vi "WSVCAP SHL Host LL Set Read_Write Parameters.vi"(0 "Transaction":T1, 1 "Wait Ticks":u32, 2 "Slave Address":u8, 5 "Bytes":u8, 7 "Sub Address [U8]":u8=191 format="%.0x", 9 "Socket Mask [U64]":u64=1 format="%016x", 11 "error in (no error)":errorcluster) -> (15 "error out":errorcluster)   [LabVIEW 2012]
uses:
  Type Defs/WSVCAP SHL Transaction Enum.ctl
  Type Defs/WSVCAP SHL Top Level Control Operation Enum.ctl
  Type Defs/WSVCAP SHL State.ctl
  Type Defs/WSVCAP SHL Top Level Control Enum.ctl
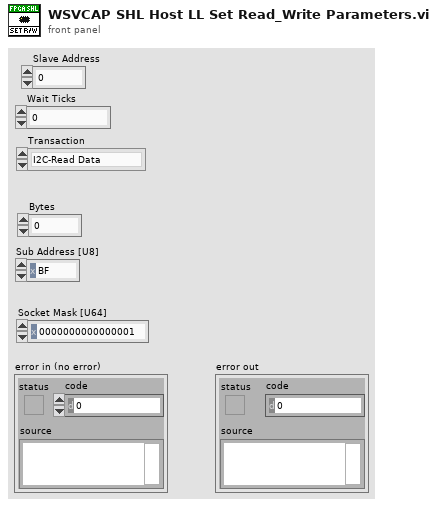
[diagram p1: front panel]
types:
  T1 = typedef "WSVCAP SHL Transaction Enum.ctl" = enum16{"I2C-Read Data", "I2C-Write Data", "SPI-Write/Read Data", "RFFE-Ext Write", "RFFE-Ext Read"}
  T2 = typedef "WSVCAP SHL Top Level Control Enum.ctl" = enum16{"Start", "Cmd", "Transaction", "Wait Ticks", "Socket Mask", "Slave Address", "Sub Address", "Bytes to Write", "Bytes to Read", "Write Data", "Write Flag", "Read Data", "Read Flag", "Ack Read", "Read Status Flag", "Ack Read Status", "Status", "Cycle Count", "Stop Cycle", "Exit"}
  T3 = typedef "WSVCAP SHL State.ctl" = enum8{"Idle", "Transfer Data"}
  T4 = typedef "WSVCAP SHL Top Level Control Operation Enum.ctl" = enum16{"Initialize", "Set Control", "Read Control", "Close"}
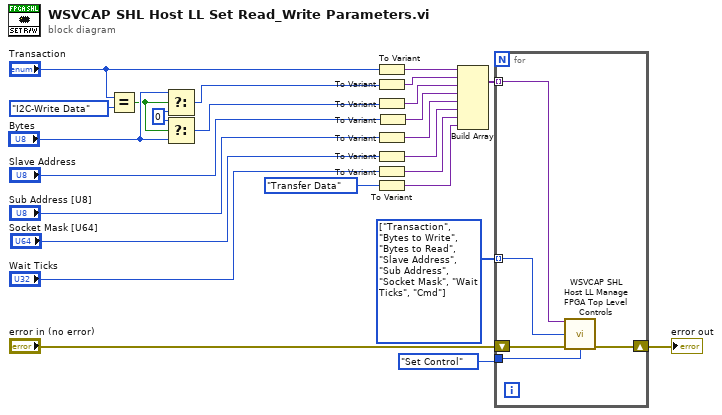
[diagram p0: block diagram]
diagram:
  w16 = u8 0 ("t")
  w18 = T2[] [enum."Transaction", enum."Bytes to Write", enum."Bytes to Read", enum."Slave Address", enum."Sub Address", enum."Socket Mask", enum."Wait Ticks", enum."Cmd"] items=["Start", "Cmd", "Transaction", "Wait Ticks", "Socket Mask", "Slave Address", "Sub Address", "Bytes to Write", "Bytes to Read", "Write Data", "Write Flag", "Read Data", "Read Flag", "Ack Read", "Read Status Flag", "Ack Read Status", "Status", "Cycle Count", "Stop Cycle", "Exit"]
  n1 = Equal?(x="Transaction", y=WSVCAP_SHL_Transaction_Enum."I2C-Write Data" ("Transaction")) -> (x = y?=w10:bool)
  n2 = Select(t="Bytes", s=w10, f=w16) -> (s? t:f=w15:u8)
  n3 = Select(t=w16, s=w10, f="Bytes") -> (s? t:f=w14:u8)
  n4 = To Variant(anything="Transaction") -> (Variant=w24:variant)
  n5 = To Variant(anything=w15) -> (Variant=w23:variant)
  n6 = To Variant(anything=w14) -> (Variant=w13:variant)
  n7 = To Variant(anything="Sub Address [U8]") -> (Variant=w9:variant)
  n8 = To Variant(anything="Socket Mask [U64]") -> (Variant=w8:variant)
  n9 = To Variant(anything="Wait Ticks") -> (Variant=w4:variant)
  n10 = To Variant(anything=WSVCAP_SHL_State."Transfer Data" ("SPI_Cmd")) -> (Variant=w19:variant)
  n11 = To Variant(anything="Slave Address") -> (Variant=w1:variant)
  n12 = Build Array(w24, w23, w13, w1, w9, w8, w4, w19) -> (w22:variant[])
  n13 = for {
    tunnel: WSVCAP_SHL_Top_Level_Control_Operation_Enum."Set Control" ("Operation") -> [w30]
    tunnel: w22 -> [w29] mode=indexing
    tunnel: w18 -> [w28] mode=indexing
    shift-right: [w26] -> w20
    shift-left: "error in (no error)" -> [w27]
    n14 = call "WSVCAP SHL Host LL Manage FPGA Top Level Controls.vi"("Value In"=w29, "FPGA Top Level Control"=w28, "error in (no error)"=w27, "Operation"=w30) -> ("error out"=w26:errorcluster)  [unwired: 10 in, 1 out]
  }
  "error out" <- w20
